vi "DrawBot.vi"(0 "picture in":picture, 1 "bot pos vector":T2, 2 "Arena Pixel Size":i16[](array[numeric])=[1000, 512], 3 "bot color":u32(colorbox)=6618880, 4 "pen":T1={"Width"=4, "Style"=enum."Solid"}) -> (5 "picture out":picture)   [LabVIEW 2015, in "MissionControl2017.lvlib" / "SubVIs - MissionControl2017.lvlib"]
uses:
  SubVIs - MissionControl2017.lvlib
  Vector.ctl
  SubVIs - Navigation2017.lvlib
  Navigation2017.lvlib
  Types - Navigation2017.lvlib
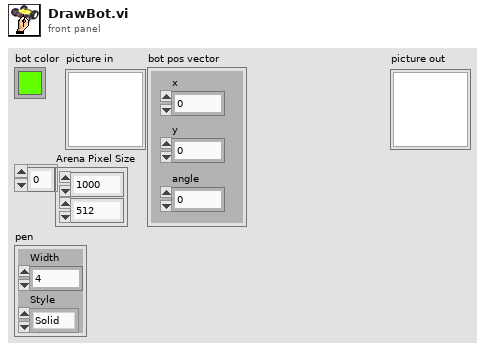
[diagram p1: front panel]
types:
  T1 = cluster{"Width":u16, "Style":enum32{"Solid", "Dash", "Dot", "DashDot", "DashDotDot"}}
  T2 = typedef "Navigation2017.lvlib/Types - Navigation2017.lvlib/Vector.ctl" = cluster{"x":dbl, "y":dbl, "angle":dbl}
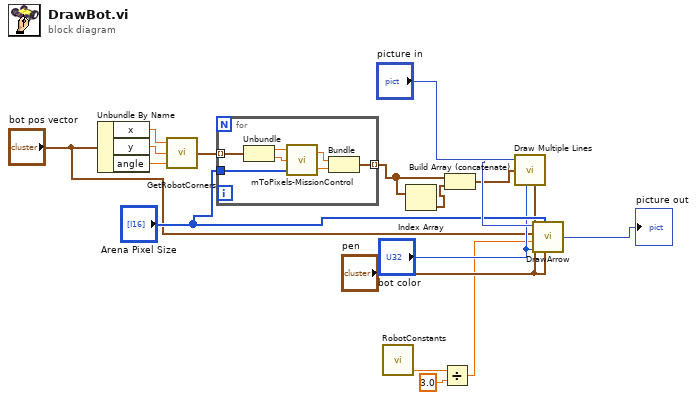
[diagram p0: block diagram]
diagram:
  n1 = Unbundle By Name("bot pos vector") -> ("x"=w17:dbl, "y"=w16:dbl, "angle"=w15:dbl)
  n2 = call "GetRobotCorners.vi"("botAngle (rad)"=w15, "botY (m)"=w16, "botX (m)"=w17) -> ("Corner Points (m)"=w14:cluster{dbl, dbl}[])
  n3 = for {
    tunnel: w14 -> [w21] mode=indexing
    tunnel: [w22] -> w1 mode=indexing
    tunnel: "Arena Pixel Size" -> [w18]
    n4 = Unbundle(w21) -> (w20:dbl, w19:dbl)
    n5 = call "mToPixels-MissionControl.vi"("Arena Pixel Dim"=w18, "y (m)"=w19, "x (m)"=w20) -> ("y (pixels)"=w23:dbl, "x (pixels)"=w24:dbl)
    n6 = Bundle("x (pixels)"=w24, "y (pixels)"=w23) -> (w22:cluster{"x (pixels)":dbl, "y (pixels)":dbl})  [unwired: 1 in]
  }
  n7 = call "RobotConstants.vi"() -> ("Robot Length (m)"=w6:dbl)  [unwired: 4 out]
  n8 = Index Array(array=w1) -> (element=w2:cluster{"x (pixels)":dbl, "y (pixels)":dbl})  [unwired: 1 in]
  n9 = Divide(x=w6, y=3.0) -> (x/y=w4:dbl)
  n10 = Build Array (concatenate)(w1, w2) -> (w3:cluster{"x (pixels)":dbl, "y (pixels)":dbl}[])
  n11 = call <vilib>:"Draw Multiple Lines.vi"("picture"="picture in", "line endpoints"=w3, "color(black)"="bot color", "pen"="pen") -> ("new picture"=w11:picture)  [unwired: 5 in]
  n12 = call "DrawArrow.vi"("Pen Style"="pen", "Arena Pixel Dim"="Arena Pixel Size", "Color"="bot color", "Length (m)"=w4, "Vector (m)"="bot pos vector", "picture"=w11) -> ("new picture"=→"picture out":picture)
